vi "ex15-1.vi"() -> ()   [LabVIEW 2013]
uses:
  <vilib>/University of Leeds/Kinesthesia Toolkit for Microsoft Kinect/_Polymorphic Configure/Event-Depth and Video.vi
  <vilib>/University of Leeds/Kinesthesia Toolkit for Microsoft Kinect/_Polymorphic Close/Close-Depth and Video.vi
  <vilib>/University of Leeds/Kinesthesia Toolkit for Microsoft Kinect/_Polymorphic Read/Read-Depth and Video.vi
panel:
  in  "stop":bool
  out "Depth picture":picture
  out "Colour picture":picture
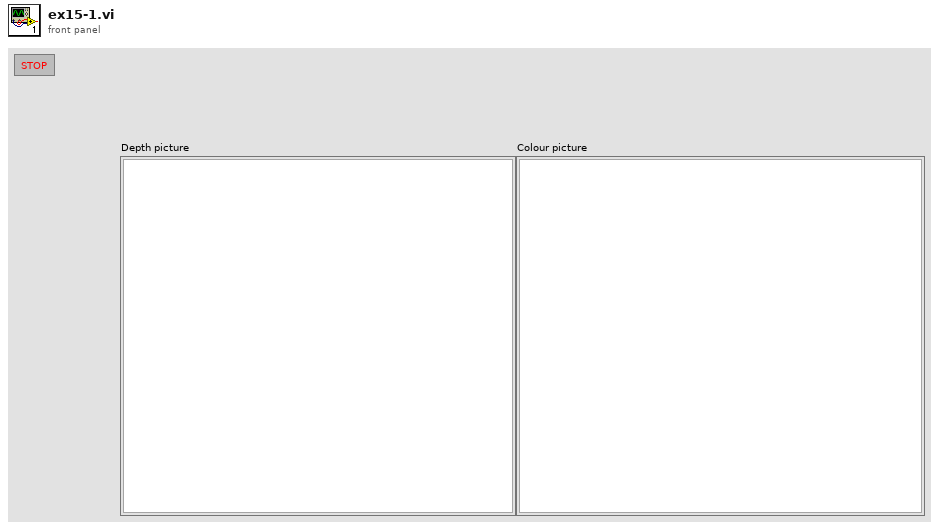
[diagram p1: front panel]
types:
  T1 = cluster{cluster{"reference out":refnum<k24>, "KinectSensors":refnum<k24>}, "get_Item":refnum<k24>}
  T2 = cluster{"reference out":refnum<k24>, "KinectSensors":refnum<k24>, "DepthStream":refnum<k24>, "ColorStream":refnum<k24>, "get_Item":refnum<k24>}
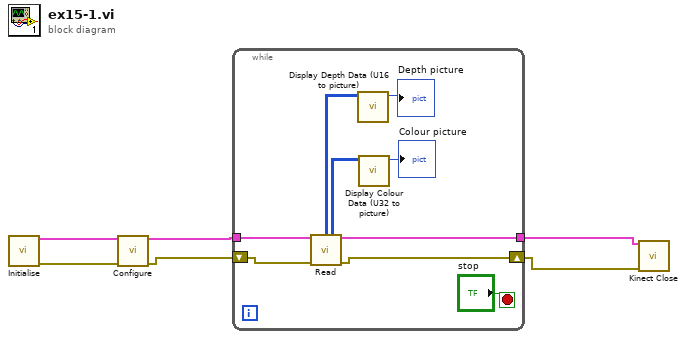
[diagram p0: block diagram]
diagram:
  n1 = call <vilib>:"Initialise.vi"() -> ("Kinect References out"=w6:T1, "error out"=w4:errorcluster)  [unwired: 14 in]
  n2 = call-poly <vilib>:"Configure.vi"("Kinect References in"=w6, "error in"=w4) -> ("Kinect References out"=w5:T2, "error out"=w3:errorcluster)  [unwired: 12 in]
  n3 = while {
    tunnel: w5 -> [w15]
    shift-right: [w8] -> w2
    shift-left: w3 -> [w9]
    tunnel: [w7] -> w1
    stop <- "stop" stop-if-true
    n4 = call-poly <vilib>:"Read.vi"("Kinect References in"=w15, "error in (no error)"=w9) -> ("Depth output array (U16)"=w11:u16[][], "Colour output array (U24, RGB)"=w12:u32[][], "Kinect References out"=w7:T2, "error out"=w8:errorcluster)  [unwired: 9 in, 1 out]
    n5 = call <vilib>:"Display Depth Data (U16 to picture).vi"("Depth output array (U16)"=w11) -> ("new picture"=→"Depth picture":picture)  [unwired: 10 in]
    n6 = call <vilib>:"Display Colour Data (U32 to picture).vi"("Colour output array (U24, RGB)"=w12) -> ("new picture"=→"Colour picture":picture)  [unwired: 10 in]
  }
  n7 = call-poly <vilib>:"Kinect Close.vi"("Kinect References in"=w1, "error  in"=w2) -> ()  [unwired: 13 in, 1 out]
